vi "Device  settings.vi"(8 "error in":errorcluster, 11 "Communication Channel":T1) -> (0 "error out":errorcluster)   [LabVIEW 2011]
uses:
  Modules/Hardware/NMR/Communication Channel.ctl
  Modules/Hardware/NMR/NMR.lvclass
panel:
  in  "stop":bool
  in  "VISA resource name":refnum<visa-resource-name>="COM16"
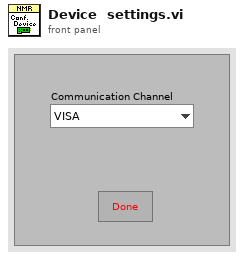
[diagram p1: front panel]
types:
  T1 = typedef "NMR.lvclass/Communication Channel.ctl" = enum16{"VISA", "DLL"}
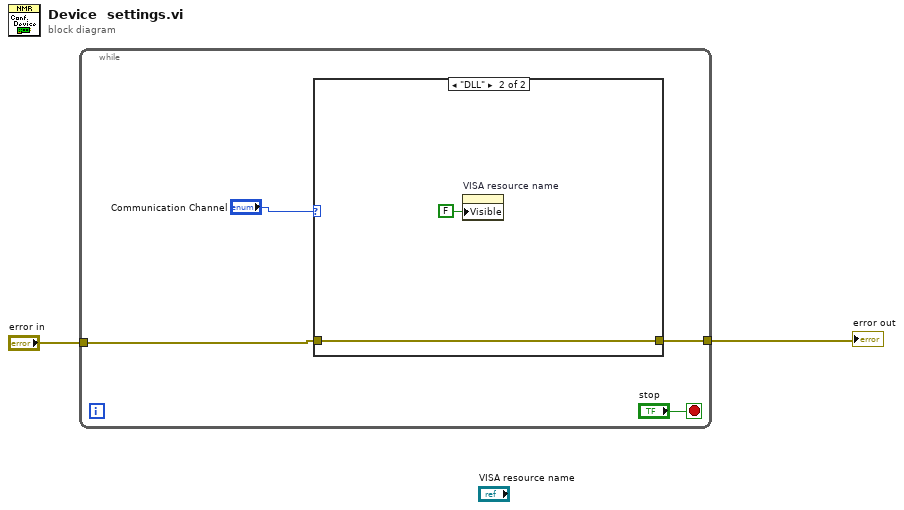
[diagram p0: block diagram]
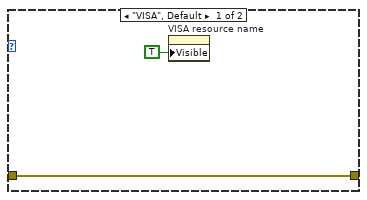
[diagram p2: hidden frame]
diagram:
  n1 = while {
    tunnel: "error in" -> [w6]
    tunnel: [w4] -> w1
    stop <- "stop" stop-if-true
    n2 = case shown="\"DLL\"" "Communication Channel" {
      tunnel: w6 -> [w7 w9]
      tunnel: [w7 w9] -> w4
      frame "VISA", Default {
        n3 = property on="VISA resource name" class="VISAName"("Visible"=TRUE) -> ()  [unwired: 2 in, 2 out]
      }
      frame "DLL" {
        n4 = property on="VISA resource name" class="VISAName"("Visible"=FALSE) -> ()  [unwired: 2 in, 2 out]
      }
    }
  }
  "error out" <- w1
